vi "三种隧道.vi"() -> ()   [LabVIEW 2013]
panel:
  out "随机数数组":dbl[](array[numeric])
  out "最大值":dbl
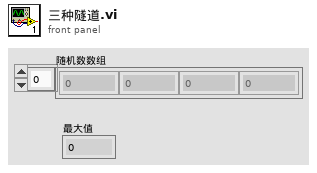
[diagram p1: front panel]
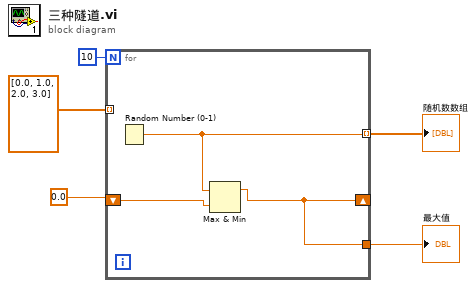
[diagram p0: block diagram]
diagram:
  n1 = for {
    N: 10 -> [_]
    tunnel: dbl[] [0.0, 1.0, 2.0, 3.0] -> [_] mode=indexing
    shift-right: [w7] -> _
    shift-left: 0.0 -> [w8]
    tunnel: [w7] -> w2
    tunnel: [w6] -> w1 mode=indexing
    n2 = Random Number (0-1)() -> (number: 0 to 1=w6:dbl)
    n3 = Max & Min(x=w6, y=w8) -> (max(x,y)=w7:dbl)  [unwired: 1 out]
  }
  "最大值" <- w2
  "随机数数组" <- w1
